vi "Facial Recognition.vi"() -> ()   [LabVIEW 2014]
uses:
  <vilib>/userdefined/High Color/IMAQdx.ctl
  <vilib>/vision/driver/NI_Vision_Acquisition_Software.lvlib
  <vilib>/vision/NI_Vision_Development_Module.lvlib
panel:
  in  "?":enum32{"基于肤色的简单人脸识别"}(tab)
  out "Session Out":T1
  in  "停止":bool
  out "?":T2(plugin-control)
  in  "?":enum32{"摄像头", "载入图片"}(radio)
  # "选择图像采集模式"
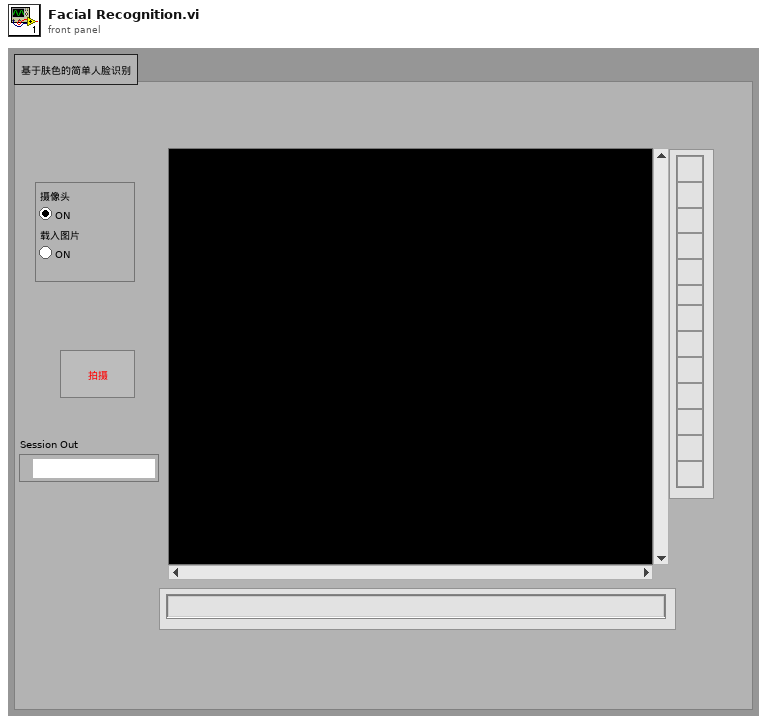
[diagram p1: front panel]
types:
  T1 = typedef "IMAQdx.ctl" = refnum<k21>
  T2 = typedef "IMAQ Image.ctl" = refnum<image>
  T3 = typedef "Particle Parameters" = i32
  T4 = cluster{"Measurement Parameter":T3, "Range Lower Value":dbl, "Range Upper Value":dbl, "Range":bool, "Measurement Type":bool}[]
  T5 = cluster{"Brightness":sgl, "Contrast":sgl, "Gamma":sgl}
  T6 = typedef "Image Type" = u32
  T7 = cluster{"Area":dbl, "Number of Holes":dbl, "Bounding Rect":cluster{"Left":dbl, "Top":dbl, "Right":dbl, "Bottom":dbl}, "Center of Mass":cluster{"X":dbl, "Y":dbl}, "Orientation":dbl, "Dimensions":cluster{"Width":dbl, "Height":dbl}}[]
  T8 = cluster{"Particle Reports (Pixels)[0]":cluster{"Area":dbl, "Number of Holes":dbl, "Bounding Rect":cluster{"Left":dbl, "Top":dbl, "Right":dbl, "Bottom":dbl}, "Center of Mass":cluster{"X":dbl, "Y":dbl}, "Orientation":dbl, "Dimensions":cluster{"Width":dbl, "Height":dbl}}, "Particle Reports (Pixels)[1]":cluster{"Area":dbl, "Number of Holes":dbl, "Bounding Rect":cluster{"Left":dbl, "Top":dbl, "Right":dbl, "Bottom":dbl}, "Center of Mass":cluster{"X":dbl, "Y":dbl}, "Orientation":dbl, "Dimensions":cluster{"Width":dbl, "Height":dbl}}, "Particle Reports (Pixels)[2]":cluster{"Area":dbl, "Number of Holes":dbl, "Bounding Rect":cluster{"Left":dbl, "Top":dbl, "Right":dbl, "Bottom":dbl}, "Center of Mass":cluster{"X":dbl, "Y":dbl}, "Orientation":dbl, "Dimensions":cluster{"Width":dbl, "Height":dbl}}, "Particle Reports (Pixels)[3]":cluster{"Area":dbl, "Number of Holes":dbl, "Bounding Rect":cluster{"Left":dbl, "Top":dbl, "Right":dbl, "Bottom":dbl}, "Center of Mass":cluster{"X":dbl, "Y":dbl}, "Orientation":dbl, "Dimensions":cluster{"Width":dbl, "Height":dbl}}, "Particle Reports (Pixels)[4]":cluster{"Area":dbl, "Number of Holes":dbl, "Bounding Rect":cluster{"Left":dbl, "Top":dbl, "Right":dbl, "Bottom":dbl}, "Center of Mass":cluster{"X":dbl, "Y":dbl}, "Orientation":dbl, "Dimensions":cluster{"Width":dbl, "Height":dbl}}, "Particle Reports (Pixels)[5]":cluster{"Area":dbl, "Number of Holes":dbl, "Bounding Rect":cluster{"Left":dbl, "Top":dbl, "Right":dbl, "Bottom":dbl}, "Center of Mass":cluster{"X":dbl, "Y":dbl}, "Orientation":dbl, "Dimensions":cluster{"Width":dbl, "Height":dbl}}, "Particle Reports (Pixels)[6]":cluster{"Area":dbl, "Number of Holes":dbl, "Bounding Rect":cluster{"Left":dbl, "Top":dbl, "Right":dbl, "Bottom":dbl}, "Center of Mass":cluster{"X":dbl, "Y":dbl}, "Orientation":dbl, "Dimensions":cluster{"Width":dbl, "Height":dbl}}, "Particle Reports (Pixels)[7]":cluster{"Area":dbl, "Number of Holes":dbl, "Bounding Rect":cluster{"Left":dbl, "Top":dbl, "Right":dbl, "Bottom":dbl}, "Center of Mass":cluster{"X":dbl, "Y":dbl}, "Orientation":dbl, "Dimensions":cluster{"Width":dbl, "Height":dbl}}, "Particle Reports (Pixels)[8]":cluster{"Area":dbl, "Number of Holes":dbl, "Bounding Rect":cluster{"Left":dbl, "Top":dbl, "Right":dbl, "Bottom":dbl}, "Center of Mass":cluster{"X":dbl, "Y":dbl}, "Orientation":dbl, "Dimensions":cluster{"Width":dbl, "Height":dbl}}}
  T9 = cluster{"Left":dbl, "Top":dbl, "Right":dbl, "Bottom":dbl}
  T10 = cluster{"Type":u32, "Version":u32, "Flags":u32, "SerialNumberHigh":u32, "SerialNumberLow":u32, "BusType":u32, "InterfaceName":string, "VendorName":string, "ModelName":string, "CameraFileName":string, "CameraAttributeURL":string}[]
  T11 = cluster{"Type":u32, "Version":u32, "Flags":u32, "SerialNumberHigh":u32, "SerialNumberLow":u32, "BusType":u32, "InterfaceName":string, "VendorName":string, "ModelName":string, "CameraFileName":string, "CameraAttributeURL":string}
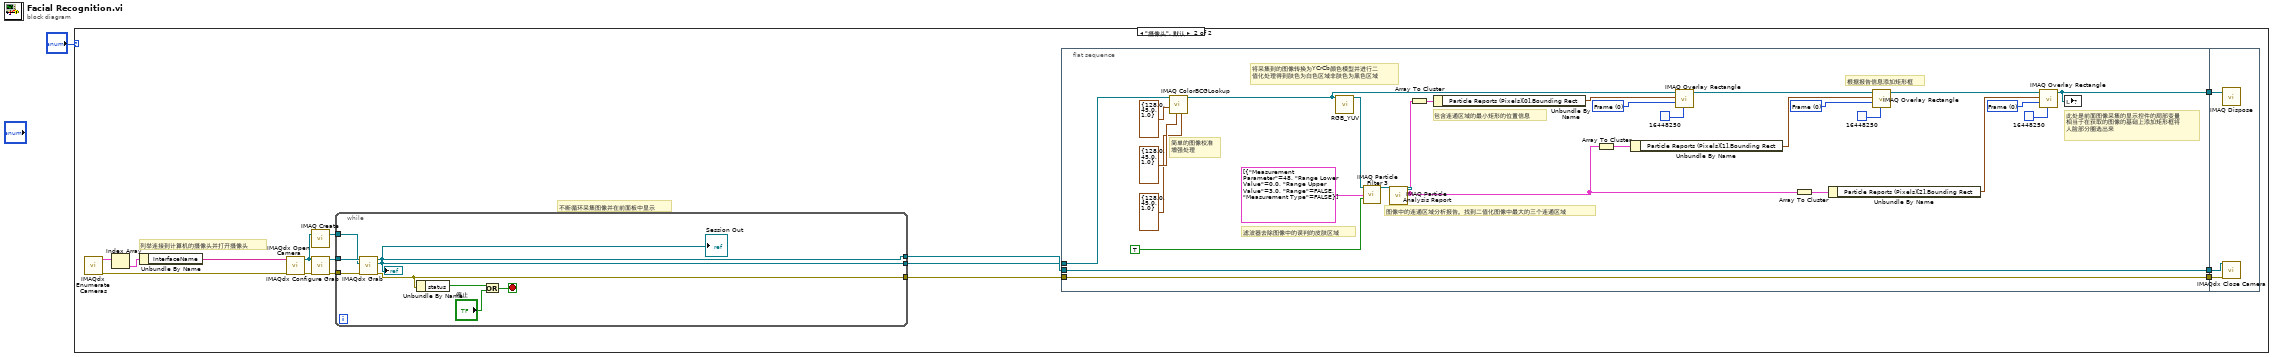
[diagram p0: block diagram]
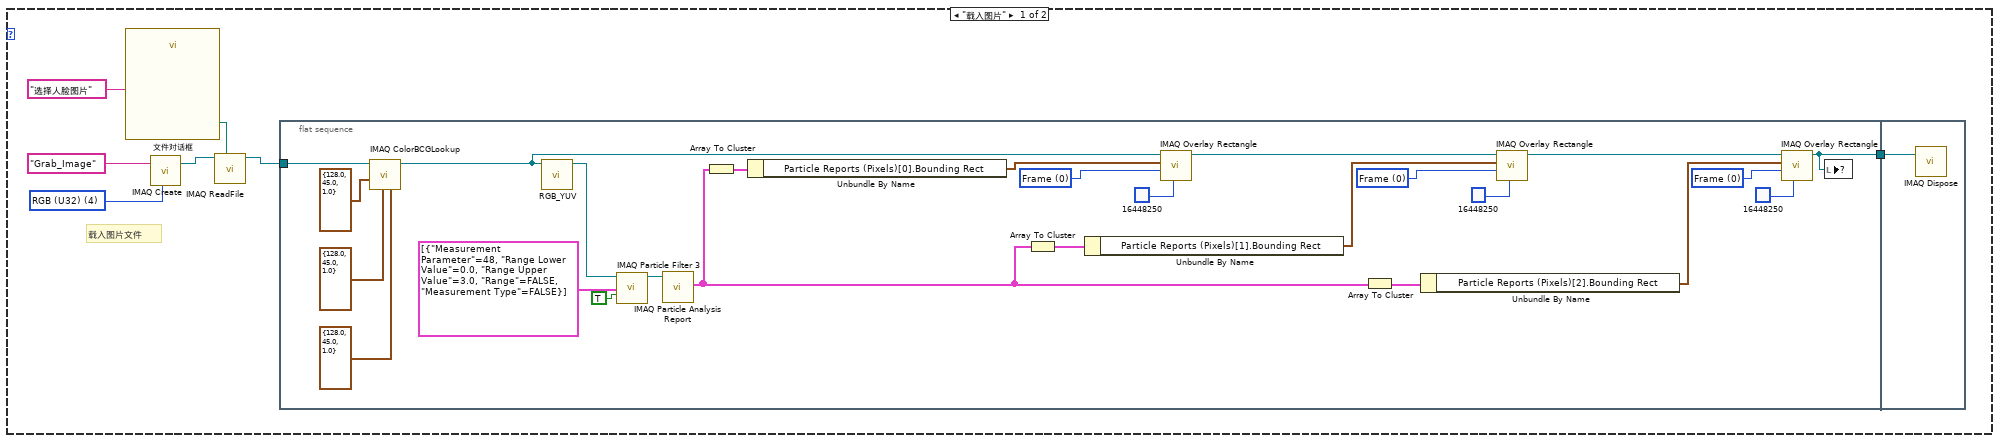
[diagram p2: hidden frame]
diagram:
  n1 = case shown="\"摄像头\", 默认" "?" {
    frame "载入图片" {
      w7 = T6 4 items=["Grayscale (U8)", "Grayscale (I16)", "Grayscale (SGL)", "Complex (CSG)", "RGB (U32)", "HSL (U32)", "RGB (U64)", "Grayscale (U16)"] ("Image Type")
      # "载入图片文件"
      n2 = call "文件对话框"("prompt"="选择人脸图片") -> ("selected path"=w4:path)  [unwired: 11 in, 3 out]
      n3 = call "IMAQ Create"("Image Name"="Grab_Image", "Image Type"=w7) -> ("New Image"=w5:T2)  [unwired: 3 in, 1 out]
      n4 = call "IMAQ ReadFile"("File Path"=w4, "Image"=w5) -> ("Image Out"=w2:T2)  [unwired: 3 in, 6 out]
      n5 = flat-sequence {
        tunnel: [w9] -> w3
        tunnel: w2 -> [w12]
        tunnel: w3 -> [w34]
        frame #0 {
          w15 = u32 0 items=["Frame", "Fill", "Highlight"] ("Drawing Mode (Frame)")
          w16 = u32 0 items=["Frame", "Fill", "Highlight"] ("Drawing Mode (Frame)")
          w24 = u32 0 items=["Frame", "Fill", "Highlight"] ("Drawing Mode (Frame)")
          n6 = call "IMAQ ColorBCGLookup"("Blue BCG Values"=T5 {"Brightness"=128.0, "Contrast"=45.0, "Gamma"=1.0}, "Green BCG Values"=T5 {"Brightness"=128.0, "Contrast"=45.0, "Gamma"=1.0}, "Red BCG Values"=T5 {"Brightness"=128.0, "Contrast"=45.0, "Gamma"=1.0}, "Image Src"=w12) -> ("Image Dst Out"=w10:T2)  [unwired: 3 in, 4 out]
          n7 = call "RGB_YUV.vi"("Image In"=w10) -> ("Image Out"=w11:T2)  [unwired: 10 in]
          n8 = call "IMAQ Particle Filter 3"("Image Src"=w11, "Selection Values"=T4 [{"Measurement Parameter"=48, "Range Lower Value"=0.0, "Range Upper Value"=3.0, "Range"=FALSE, "Measurement Type"=FALSE}], "Keep/Remove Particles (F)"=TRUE) -> ("Image Dst Out"=w28:T2)  [unwired: 10 in, 2 out]
          n9 = call "IMAQ Particle Analysis Report"("Image"=w28) -> ("Particle Reports (Pixels)"=w21:T7)  [unwired: 5 in, 5 out]
          n10 = Array To Cluster(array=w21) -> (cluster=w27:T8)
          n11 = Unbundle By Name(w27) -> ("Particle Reports (Pixels)[0].Bounding Rect"=w26:T9)
          n12 = Array To Cluster(array=w21) -> (cluster=w23:T8)
          n13 = Unbundle By Name(w23) -> ("Particle Reports (Pixels)[1].Bounding Rect"=w14:T9)
          n14 = call "IMAQ Overlay Rectangle"("Color"=u32 16448250, "Drawing Mode (Frame)"=w24, "Rectangle"=w26, "Image"=w10) -> ("Image Out"=w18:T2)  [unwired: 6 in, 1 out]
          n15 = Array To Cluster(array=w21) -> (cluster=w22:T8)
          n16 = Unbundle By Name(w22) -> ("Particle Reports (Pixels)[2].Bounding Rect"=w13:T9)
          n17 = call "IMAQ Overlay Rectangle"("Color"=u32 16448250, "Drawing Mode (Frame)"=w16, "Rectangle"=w14, "Image"=w18) -> ("Image Out"=w17:T2)  [unwired: 6 in, 1 out]
          n18 = call "IMAQ Overlay Rectangle"("Color"=u32 16448250, "Drawing Mode (Frame)"=w15, "Rectangle"=w13, "Image"=w17) -> ("Image Out"=w9:T2)  [unwired: 6 in, 1 out]
          n19 = local write item#2(w9) -> ()
        }
        frame #1 {
          n20 = call "IMAQ Dispose"("Image"=w34) -> ()  [unwired: 5 in, 1 out]
        }
      }
    }
    frame "摄像头", Default {
      # "不断循环采集图像并在前面板中显示"
      # "列举连接到计算机的摄像头并打开摄像头"
      n21 = call <vilib>:"IMAQdx Enumerate Cameras.vi"() -> ("error out"=w43:errorcluster, "Camera Information Array"=w46:T10)  [unwired: 10 in]
      n22 = Index Array(array=w46) -> (element=w45:T11)  [unwired: 1 in]
      n23 = Unbundle By Name(w45) -> ("InterfaceName"=w44:string)
      n24 = call <vilib>:"IMAQdx Open Camera.vi"("error in"=w43, "Session In"=w44) -> ("error out"=w42:errorcluster, "Session Out"=w40:T1)  [unwired: 8 in]
      n25 = call "IMAQ Create"("Image Name"=w40) -> ("New Image"=w39:T2)  [unwired: 4 in, 1 out]
      n26 = call <vilib>:"IMAQdx Configure Grab.vi"("error in"=w42, "Session In"=w40) -> ("error out"=w38:errorcluster, "Session Out"=w41:T1)  [unwired: 8 in]
      n27 = while {
        tunnel: [w83] -> w37
        tunnel: w41 -> [w88]
        tunnel: w39 -> [w87]
        tunnel: w38 -> [w86]
        tunnel: [w81] -> w36
        tunnel: [w80] -> w35
        stop <- w85 stop-if-true
        n28 = call <vilib>:"IMAQdx Grab.vi"("error in"=w86, "Image In"=w87, "Session In"=w88) -> ("error out"=w83:errorcluster, "Image Out"=w80:T2, "Session Out"=w81:T1)  [unwired: 5 in, 1 out]
        "Session Out" <- w81
        "?" <- w80
        n29 = Unbundle By Name(w83) -> ("status"=w82:bool)
        n30 = Or(x=w82, y="停止") -> (x .or. y?=w85:bool)
      }
      n31 = flat-sequence {
        tunnel: w37 -> [w55]
        tunnel: [w55] -> w49
        tunnel: [w54] -> w48
        tunnel: [w51] -> w47
        tunnel: w36 -> [w54]
        tunnel: w35 -> [w50]
        tunnel: w49 -> [w77]
        tunnel: w48 -> [w78]
        tunnel: w47 -> [w79]
        frame #0 {
          w58 = u32 0 items=["Frame", "Fill", "Highlight"] ("Drawing Mode (Frame)")
          w59 = u32 0 items=["Frame", "Fill", "Highlight"] ("Drawing Mode (Frame)")
          w67 = u32 0 items=["Frame", "Fill", "Highlight"] ("Drawing Mode (Frame)")
          # "此处是前面图像采集的显示控件的局部变量\n相当于在获取的图像的基础上添加矩形框将\n人脸部分圈选出来"
          # "根据报告信息添加矩形框"
          # "包含连通区域的最小矩形的位置信息"
          # "图像中的连通区域分析报告。找到二值化图像中最大的三个连通区域"
          # "滤波器去除图像中的误判的皮肤区域"
          # "简单的图像校准\n增强处理"
          # "将采集到的图像转换为YCrCb颜色模型并进行二\n值化处理得到肤色为白色区域非肤色为黑色区域"
          n32 = call "IMAQ ColorBCGLookup"("Blue BCG Values"=T5 {"Brightness"=128.0, "Contrast"=45.0, "Gamma"=1.0}, "Green BCG Values"=T5 {"Brightness"=128.0, "Contrast"=45.0, "Gamma"=1.0}, "Red BCG Values"=T5 {"Brightness"=128.0, "Contrast"=45.0, "Gamma"=1.0}, "Image Src"=w50) -> ("Image Dst Out"=w53:T2)  [unwired: 3 in, 4 out]
          n33 = call "RGB_YUV.vi"("Image In"=w53) -> ("Image Out"=w52:T2)  [unwired: 10 in]
          n34 = call "IMAQ Particle Filter 3"("Image Src"=w52, "Selection Values"=T4 [{"Measurement Parameter"=48, "Range Lower Value"=0.0, "Range Upper Value"=3.0, "Range"=FALSE, "Measurement Type"=FALSE}], "Keep/Remove Particles (F)"=TRUE) -> ("Image Dst Out"=w71:T2)  [unwired: 10 in, 2 out]
          n35 = call "IMAQ Particle Analysis Report"("Image"=w71) -> ("Particle Reports (Pixels)"=w64:T7)  [unwired: 5 in, 5 out]
          n36 = Array To Cluster(array=w64) -> (cluster=w70:T8)
          n37 = Unbundle By Name(w70) -> ("Particle Reports (Pixels)[0].Bounding Rect"=w69:T9)
          n38 = Array To Cluster(array=w64) -> (cluster=w66:T8)
          n39 = Unbundle By Name(w66) -> ("Particle Reports (Pixels)[1].Bounding Rect"=w57:T9)
          n40 = call "IMAQ Overlay Rectangle"("Color"=u32 16448250, "Drawing Mode (Frame)"=w67, "Rectangle"=w69, "Image"=w53) -> ("Image Out"=w61:T2)  [unwired: 6 in, 1 out]
          n41 = Array To Cluster(array=w64) -> (cluster=w65:T8)
          n42 = Unbundle By Name(w65) -> ("Particle Reports (Pixels)[2].Bounding Rect"=w56:T9)
          n43 = call "IMAQ Overlay Rectangle"("Color"=u32 16448250, "Drawing Mode (Frame)"=w59, "Rectangle"=w57, "Image"=w61) -> ("Image Out"=w60:T2)  [unwired: 6 in, 1 out]
          n44 = call "IMAQ Overlay Rectangle"("Color"=u32 16448250, "Drawing Mode (Frame)"=w58, "Rectangle"=w56, "Image"=w60) -> ("Image Out"=w51:T2)  [unwired: 6 in, 1 out]
          n45 = local write item#2(w51) -> ()
        }
        frame #1 {
          n46 = call "IMAQ Dispose"("Image"=w79) -> ()  [unwired: 5 in, 1 out]
          n47 = call <vilib>:"IMAQdx Close Camera.vi"("error in"=w77, "Session In"=w78) -> ()  [unwired: 9 in, 1 out]
        }
      }
    }
  }
